vi "PS Comm Globals.vi"() -> ()   [LabVIEW 2021]
panel:
  in  "Max Slew [A/S]":dbl format="%.1f"
  in  "Max Current [kA]":dbl format="%.2f"
  in  "B=F(I)":dbl[](array[numeric])=[0.0, 1.0, 0.0] format="%.5e"
  in  "I=F(B)":dbl[](array[numeric])=[0.0, 1.0, 0.0] format="%.5e"
  in  "PS Communication Port":refnum<visa-resource-name>
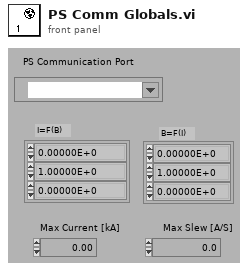
[diagram p1: front panel]
diagram:
